vi "PV ModulLine miscellaneous.vi"(8 "error in (no error)":errorcluster, 9 "PV ModulLine miscellaneous - Cluster":T1={"Parameter"=enum." Keyboard interlock (008)", "Parameter\nread only<->describe"=FALSE, "off<->on   "=TRUE, "Unit adress"=10, "SensEnable"=0} {"SensEnable" items=["OFF (default)", "ON", "A1 ( 1)", "A2 (2)", "B1 (3)", "B2 (4)", "Komplex"]; "Unit adress" min=1 max=255 step=1}, 10 "Adress of unit":u16=10 max=999 step=1, 11 "VISA session":refnum<visa-resource-name>) -> (0 "error out":errorcluster, 2 "response (data)":string, 3 "dup VISA session":refnum<visa-resource-name>)   [LabVIEW 2021, in "Pfeiffer Vacuum.lvlib"]
doc: "There are 5 parameters available, only one of which can be enabled at a time. \n\nKeyboard interlock (008)\nSensor enable (041)\nOperating hours (314)\nHardware version (354)\nUnit adress (797)\n\nNote: Any settings for an parameter that is not selected will be ignored. If a value is out of range, it will be changed to either the upper or the lower limit of the range."
uses:
  <instrlib>/Pfeiffer Vacuum/Pfeiffer Vacuum.lvlib
  <instrlib>/Pfeiffer Vacuum/Public/ModulLine/PV ModulLine miscellaneous - Cluster.ctl
panel:
  # "<------------  -----------> \n Keyboard interlock :                     OFF                          ON"
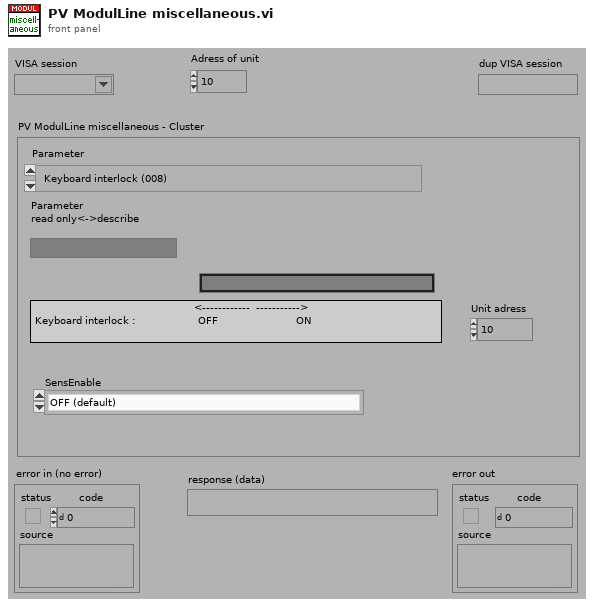
[diagram p1: front panel]
types:
  T1 = typedef "Pfeiffer Vacuum.lvlib/PV ModulLine miscellaneous - Cluster.ctl" = cluster{"Parameter":enum16{" Keyboard interlock (008)", " Sensor enable (041)", " Operating hours TPG500 (314)", " Hardware Version (354)", " Unit adress (797)"}, "Parameter\nread only<->describe":bool, "off<->on   ":bool, "Unit adress":i16, "SensEnable":u16}
  T2 = enum16{" Keyboard interlock (008)", " Sensor enable (041)", " Operating hours TPG500 (314)", " Hardware Version (354)", " Unit adress (797)"}
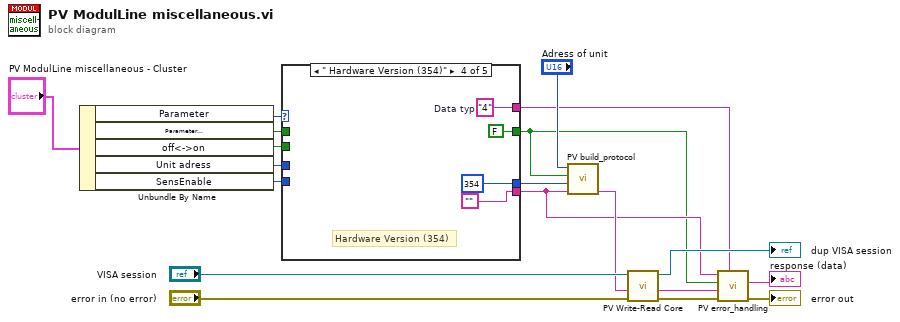
[diagram p0: block diagram]
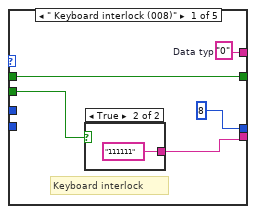
[diagram p2: hidden frame]
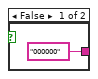
[diagram p3: hidden frame]
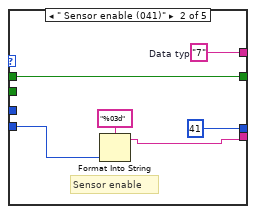
[diagram p4: hidden frame]
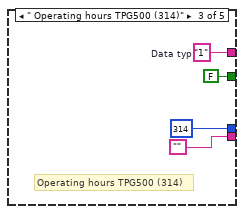
[diagram p5: hidden frame]
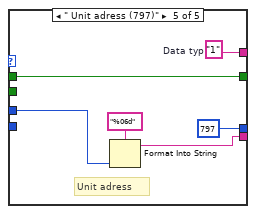
[diagram p6: hidden frame]
diagram:
  n1 = Unbundle By Name("PV ModulLine miscellaneous - Cluster") -> ("Parameter"=w17:T2, "Parameter\nread only<->describe"=w16:bool, "off<->on"=w14:bool, "Unit adress"=w13:i16, "SensEnable"=w2:u16)
  n2 = case shown="\" Hardware Version (354)\"" w17 {
    tunnel: [u16 8 ("Parameter-number") u16 41 ("Parameter-number") u16 314 ("Parameter-number") u16 354 ("Parameter-number") u16 797 ("Parameter-number")] -> w18
    tunnel: [w20 w28 "" "" w45] -> w5
    tunnel: [w22 w30 FALSE ("Parameter\nread only<->describe") FALSE ("Parameter\nread only<->describe") w43] -> w4
    tunnel: w16 -> [w22 w30 _ _ w43]
    tunnel: w14 -> [w21 _ _ _ _]
    tunnel: w13 -> [_ _ _ _ w42]
    tunnel: [w23 w31 w35 w39 w41] -> w6
    tunnel: w2 -> [_ w27 _ _ _]
    frame " Keyboard interlock (008)" {
      w23 = "0"  # Data typ
      # "Keyboard interlock"
      n3 = case shown="True" w21 {
        tunnel: ["000000" ("Data") "111111" ("Data")] -> w20
        frame False {
        }
        frame True {
        }
      }
    }
    frame " Sensor enable (041)" {
      w31 = "7"  # Data typ
      # "Sensor enable"
      n4 = Format Into String(format string="%03d" ("Format-String"), w27) -> (resulting string=w28:string)  [unwired: 2 in, 1 out]
    }
    frame " Operating hours TPG500 (314)" {
      w35 = "1"  # Data typ
      # "Operating hours TPG500 (314)"
    }
    frame " Hardware Version (354)" {
      w39 = "4"  # Data typ
      # "Hardware Version (354)"
    }
    frame " Unit adress (797)" {
      w41 = "1"  # Data typ
      # "Unit adress"
      n5 = Format Into String(format string="%06d" ("Format-String"), w42) -> (resulting string=w45:string)  [unwired: 2 in, 1 out]
    }
  }
  n6 = call <instrlib>:"PV build_protocol.vi"("Data"=w5, "Parameter-number"=w18, "parameter\nread<->describe"=w4, "Adress"="Adress of unit") -> ("output"=w10:string)  [unwired: 3 in]
  n7 = call <instrlib>:"PV Write-Read Core.vi"("error in"="error in (no error)", "Write data in"=w10, "VISA session"="VISA session") -> ("error out"=w7:errorcluster, "response (data) out"=w8:string, "dup VISA session"=→"dup VISA session":refnum<visa-resource-name>)  [unwired: 2 in]
  n8 = call <instrlib>:"PV error_handling.vi"("Data Typ in"=w6, "error in"=w7, "response (data) in"=w8, "Parameter\nread only<->describe"=w4, "data in"=w5) -> ("error out"=→"error out":errorcluster, "Data out"=→"response (data)":string)  [unwired: 4 in, 1 out]
